vi "EncoderPIDForMotorOutput.vi"(0 "RobotEncoderRef":T7, 5 "MotorIndex":T2, 7 "Target":dbl, 9 "PID gains":T1={"proportional gain (Kc)"=1.0, "integral time (Ti, min)"=0.01, "derivative time (Td, min)"=0.0} {"derivative time (Td, min)" format="%.3f"; "integral time (Ti, min)" format="%.3f"; "proportional gain (Kc)" format="%.3f"}, 11 "error in (no error)":errorcluster) -> (6 "Output":dbl, 15 "error out":errorcluster)   [LabVIEW 2013]
uses:
  <vilib>/Rock Robotics/WPI/Encoder/WPI_EncoderDevRef.ctl
  <vilib>/Rock Robotics/SystemInterfaces/Encoder/FPGA_EncoderIdx.ctl
  <vilib>/Rock Robotics/SystemInterfaces/Counter/FPGA_CounterCtrSystemIndex.ctl
  <vilib>/Rock Robotics/WPI/Encoder/WPI_EncoderType.ctl
  <vilib>/Rock Robotics/WPI/RobotDrive/WPI_RobotDriveMotorSelectorEnum.ctl
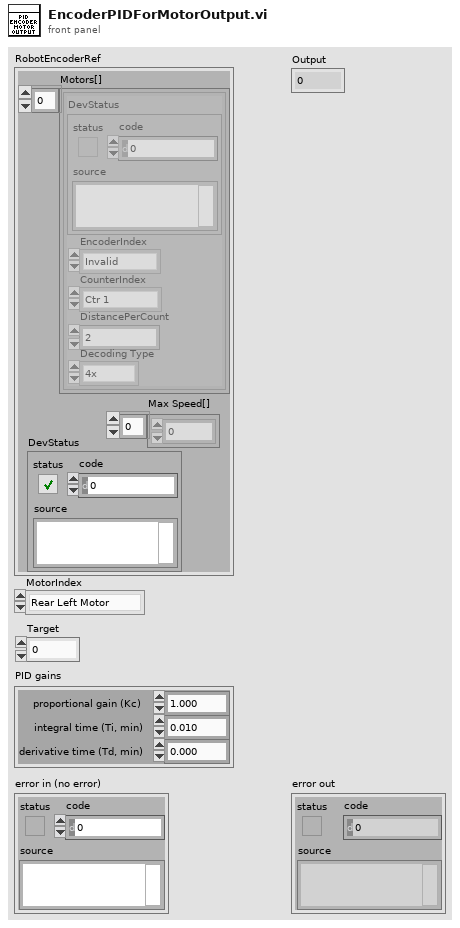
[diagram p1: front panel]
types:
  T1 = cluster{"proportional gain (Kc)":dbl, "integral time (Ti, min)":dbl, "derivative time (Td, min)":dbl}
  T2 = typedef "WPI_RobotDriveMotorSelectorEnum.ctl" = enum16{"Rear Left Motor", "Rear Right Motor", "Front Left Motor", "Front Right Motor"}
  T3 = typedef "WPI_EncoderDevRef.ctl" = cluster{"DevStatus":errorcluster, "EncoderIndex":T4, "CounterIndex":T5, "DistancePerCount":dbl, "Decoding Type":T6}
  T4 = typedef "FPGA_EncoderIdx.ctl" = enum8{"Enc 0", "Enc 1", "Enc 2", "Enc 3", "Invalid"}
  T5 = typedef "FPGA_CounterCtrSystemIndex.ctl" = enum8{"Ctr 0", "Ctr 1", "Ctr 2", "Ctr 3", "Ctr 4", "Ctr 5", "Ctr 6", "Ctr 7", "Invalid"}
  T6 = typedef "WPI_EncoderType.ctl" = enum16{"1x", "2x", "4x"}
  T7 = cluster{"Motors[]":T3[], "DevStatus":errorcluster, "Max Speed[]":dbl[]}
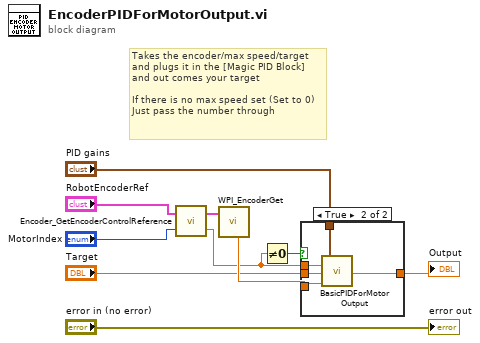
[diagram p0: block diagram]
diagram:
  # "Takes the encoder/max speed/target\nand plugs it in the [Magic PID Block]\nand out comes your target\n\nIf there is no max speed set (Set to 0)\nJust pass the number through"
  n1 = call "Encoder_GetEncoderControlReference.vi"("MotorIndex"="MotorIndex", "RobotEncoderRef"="RobotEncoderRef") -> ("Max Speed"=w1:dbl, "EncoderDevRef"=w8:T3)
  n2 = call <vilib>:"WPI_EncoderGet.vi"("EncoderDevRef"=w8) -> ("Rate"=w7:dbl)  [unwired: 5 in, 5 out]
  n3 = Not Equal To 0?(x=w1) -> (x != 0?=w2:bool)
  n4 = case shown="True" w2 {
    tunnel: w1 -> [_ w16]
    tunnel: w7 -> [_ w15]
    tunnel: "Target" -> [w11 w14]
    tunnel: "PID gains" -> [_ w13]
    tunnel: [w11 w12] -> w3
    frame False {
    }
    frame True {
      n5 = call "BasicPIDForMotorOutput.vi"("CurrentSpeed"=w15, "SetSpeed"=w14, "MaxSpeed"=w16, "PID gains"=w13) -> ("Output"=w12:dbl)
    }
  }
  "Output" <- w3
  "error out" <- "error in (no error)"
